vi "CAN_parse_motor_controller.vi"(11 "CAN message data":u8[](array[numeric])) -> ()   [LabVIEW 2018]
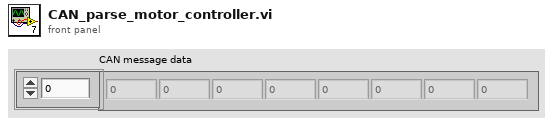
[diagram p1: front panel]
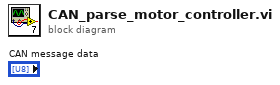
[diagram p0: block diagram]
diagram:
